vi "E_pressure_comparitor.vi"(1 "Vacuum State":bool[](array[boolean])) -> (0 "output array":bool[](array[boolean]))   [LabVIEW 2015]
panel:
  in  "Turbo Status Array":bool[](array[boolean])
  in  "Pressures":dbl[](array[numeric])
  # "Beamline 1"
  # "1"
  # "Beamline 2"
  # "2"
  # "1"
  # "3"
  # "Beamline 3"
  # "2"
  # "4"
  # "LEIL"
  # "5"
  # "3"
  # "6"
  # "Turbo 1"
  # "7"
  # "Turbo 2"
  # "8"
  # "Turbo 3"
  # "Post LEIL"
  # "Micro Ion"
  # "Cryo 1"
  # "Cryo 2"
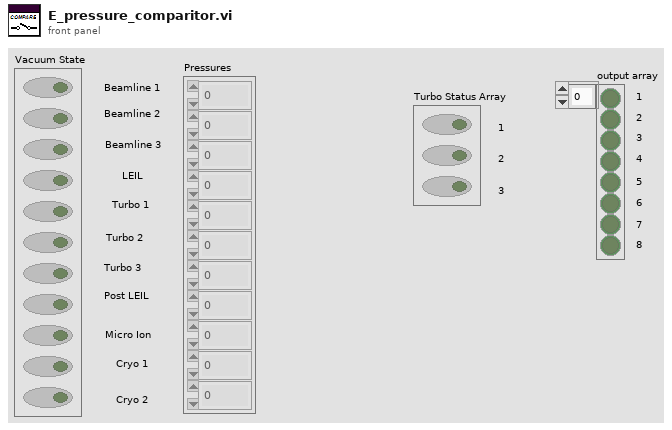
[diagram p1: front panel]
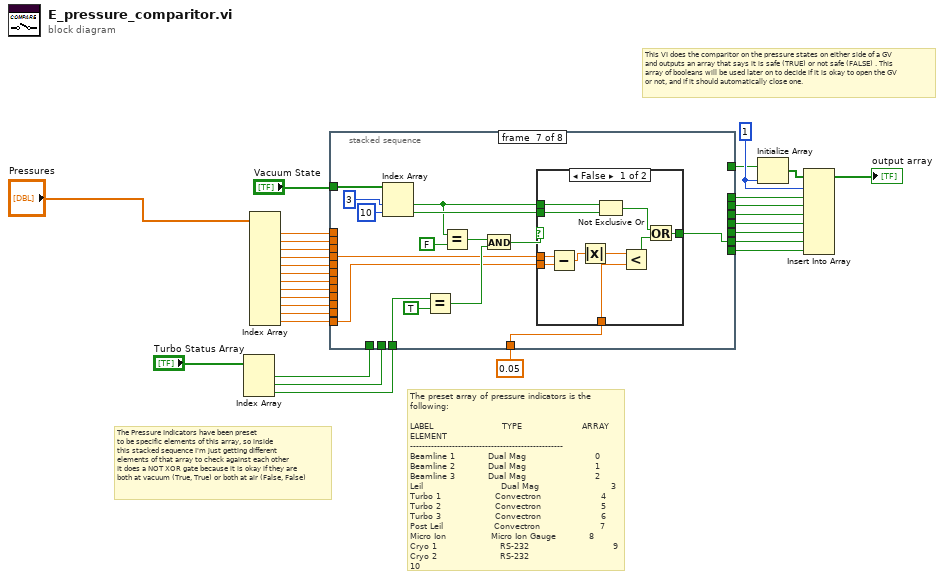
[diagram p0: block diagram]
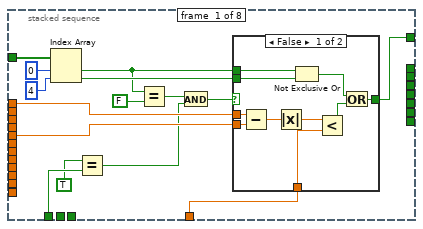
[diagram p2: hidden frame]
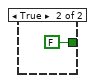
[diagram p3: hidden frame]
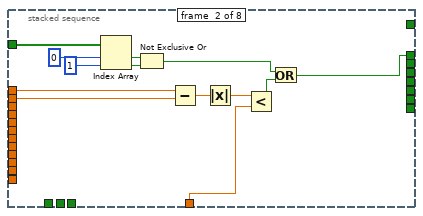
[diagram p4: hidden frame]
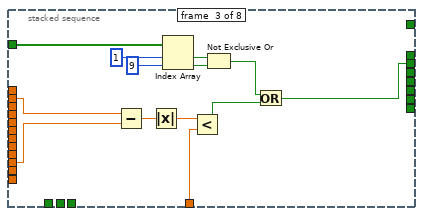
[diagram p5: hidden frame]
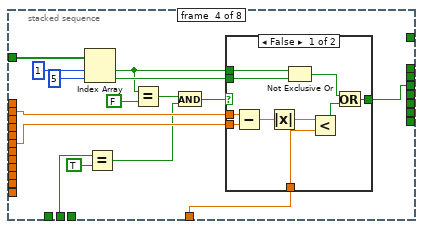
[diagram p6: hidden frame]
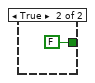
[diagram p7: hidden frame]
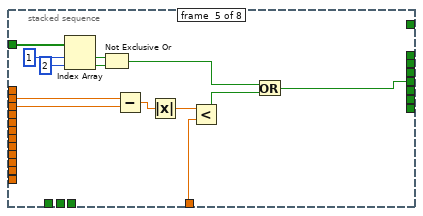
[diagram p8: hidden frame]
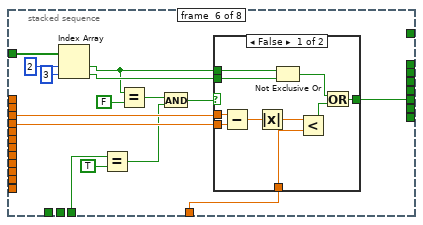
[diagram p9: hidden frame]
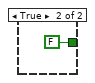
[diagram p10: hidden frame]
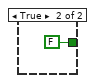
[diagram p11: hidden frame]
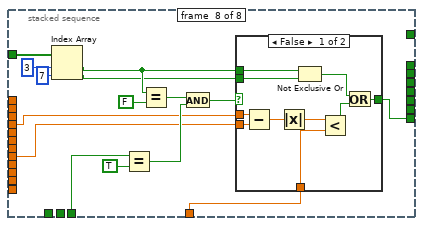
[diagram p12: hidden frame]
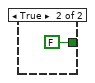
[diagram p13: hidden frame]
diagram:
  w22 = 1 ("dimension size")
  # "The preset array of pressure indicators is the following:\n\nLABEL                       TYPE                    ARRAY ELEMENT\n---------------------------------------------------\nBeamline 1           Dual Mag                       0\nBeamline 2           Dual Mag                       1\nBeamline 3           Dual Mag                       2\nLeil                          Dual Mag                        3\nTurbo 1                  Convectron                    4\nTurbo 2                  Convectron                    5\nTurbo 3                  Convectron                    6\nPost Leil                 Convectron                    7\nMicro Ion               Micro Ion Gauge           8\nCryo 1                     RS-232                            9\nCryo 2                     RS-232                            10"
  # "The Pressure Indicators have been preset\nto be specific elements of this array, so inside \nthis stacked sequence I'm just getting different\nelements of that array to check against each other \nIt does a NOT XOR gate because it is okay if they are \nboth at vacuum (True, True) or both at air (False, False)"
  # "This VI does the comparitor on the pressure states on either side of a GV\nand outputs an array that says it is safe (TRUE) or not safe (FALSE) . This\narray of booleans will be used later on to decide if it is okay to open the GV\nor not, and if it should automatically close one."
  n1 = Index Array(array="Turbo Status Array") -> (element #1=w4:bool, element #2=w3:bool, element #3=w2:bool)  [unwired: 3 in]
  n2 = Index Array(array="Pressures") -> (element #1=w17:dbl, element #2=w16:dbl, element #3=w15:dbl, element #4=w14:dbl, element #5=w13:dbl, element #6=w12:dbl, element #7=w11:dbl, element #8=w10:dbl, element #9=w9:dbl, element #10=w8:dbl, element #11=w7:dbl, element #12=w1:dbl)  [unwired: 12 in]
  n3 = stacked-sequence {
    tunnel: [_ w57 _ _ _ _ _ _] -> w29
    tunnel: [_ _ w70 _ _ _ _ _] -> w28
    tunnel: [_ _ _ w93 _ _ _ _] -> w27
    tunnel: [_ _ _ _ w109 _ _ _] -> w26
    tunnel: [_ _ _ _ _ w133 _ _] -> w25
    tunnel: [_ _ _ _ _ _ w151 _] -> w24
    tunnel: [_ _ _ _ _ _ _ w180] -> w23
    tunnel: [w36 _ _ _ _ _ _ _] -> w21
    tunnel: "Vacuum State" -> [w42 w65 w78 w95 w117 w134 w160 w186]
    tunnel: w17 -> [w41 w61 _ _ _ _ _ _]
    tunnel: w16 -> [_ w60 w74 w92 w112 _ _ _]
    tunnel: w15 -> [_ _ _ _ w111 w131 _ _]
    tunnel: w14 -> [_ _ _ _ _ w130 w153 w176]
    tunnel: w13 -> [w40 _ _ _ _ _ _ _]
    tunnel: w12 -> [_ _ _ w91 _ _ _ _]
    tunnel: w11 -> [_ _ _ _ _ _ _ _]
    tunnel: w10 -> [_ _ _ _ _ _ _ w175]
    tunnel: w9 -> [_ _ _ _ _ _ _ _]
    tunnel: w8 -> [_ _ w73 _ _ _ _ _]
    tunnel: w7 -> [_ _ _ _ _ _ _ _]
    tunnel: 0.05 ("y") -> [w39 w59 w72 w94 w113 w132 w154 w179]
    tunnel: w4 -> [w38 _ _ _ _ _ _ _]
    tunnel: w3 -> [_ _ _ w83 _ _ _ _]
    tunnel: w2 -> [_ _ _ _ _ w124 w152 w174]
    tunnel: w1 -> [_ _ _ _ _ _ w148 _]
    frame #0 {
      n4 = Index Array(array=w42, index #1=0 ("index"), index #2=4 ("index")) -> (element #1=w35:bool, element #2=w45:bool)
      n5 = Equal?(x=TRUE ("y"), y=w38) -> (x = y?=w32:bool)
      n6 = Equal?(x=w35, y=FALSE) -> (x = y?=w33:bool)
      n7 = And(x=w33, y=w32) -> (x .and. y?=w31:bool)
      n8 = case shown="False" w31 {
        tunnel: w35 -> [w55 _]
        tunnel: w45 -> [w54 _]
        tunnel: w41 -> [w53 _]
        tunnel: w40 -> [w52 _]
        tunnel: [w47 FALSE] -> w36
        tunnel: w39 -> [w46 _]
        frame False {
          n9 = Subtract(x=w53, y=w52) -> (x-y=w51:dbl)
          n10 = Absolute Value(x=w51) -> (abs(x)=w50:dbl)
          n11 = Not Exclusive Or(1:w54, 2:w55) -> (0:w48:bool)
          n12 = Less?(x=w50, y=w46) -> (x < y?=w49:bool)
          n13 = Or(x=w48, y=w49) -> (x .or. y?=w47:bool)
        }
        frame True {
        }
      }
    }
    frame #1 {
      n14 = Index Array(array=w65, index #1=0 ("index"), index #2=1 ("index")) -> (element #1=w69:bool, element #2=w68:bool)
      n15 = Not Exclusive Or(1:w68, 2:w69) -> (0:w58:bool)
      n16 = Subtract(x=w61, y=w60) -> (x-y=w64:dbl)
      n17 = Absolute Value(x=w64) -> (abs(x)=w63:dbl)
      n18 = Less?(x=w63, y=w59) -> (x < y?=w62:bool)
      n19 = Or(x=w58, y=w62) -> (x .or. y?=w57:bool)
    }
    frame #2 {
      n20 = Subtract(x=w74, y=w73) -> (x-y=w77:dbl)
      n21 = Absolute Value(x=w77) -> (abs(x)=w76:dbl)
      n22 = Index Array(array=w78, index #1=1 ("index"), index #2=9 ("index")) -> (element #1=w82:bool, element #2=w81:bool)
      n23 = Less?(x=w76, y=w72) -> (x < y?=w75:bool)
      n24 = Not Exclusive Or(1:w81, 2:w82) -> (0:w71:bool)
      n25 = Or(x=w71, y=w75) -> (x .or. y?=w70:bool)
    }
    frame #3 {
      n26 = Index Array(array=w95, index #1=1 ("index"), index #2=5 ("index")) -> (element #1=w86:bool, element #2=w90:bool)
      n27 = Equal?(x=w83, y=TRUE) -> (x = y?=w84:bool)
      n28 = Equal?(x=w86, y=FALSE) -> (x = y?=w88:bool)
      n29 = And(x=w88, y=w84) -> (x .and. y?=w87:bool)
      n30 = case shown="False" w87 {
        tunnel: w86 -> [w107 _]
        tunnel: w90 -> [w106 _]
        tunnel: w92 -> [w105 _]
        tunnel: w91 -> [w104 _]
        tunnel: [w99 FALSE] -> w93
        tunnel: w94 -> [w98 _]
        frame False {
          n31 = Subtract(x=w105, y=w104) -> (x-y=w103:dbl)
          n32 = Absolute Value(x=w103) -> (abs(x)=w102:dbl)
          n33 = Not Exclusive Or(1:w106, 2:w107) -> (0:w100:bool)
          n34 = Less?(x=w102, y=w98) -> (x < y?=w101:bool)
          n35 = Or(x=w100, y=w101) -> (x .or. y?=w99:bool)
        }
        frame True {
        }
      }
    }
    frame #4 {
      n36 = Index Array(array=w117, index #1=1 ("index"), index #2=2 ("index")) -> (element #1=w121:bool, element #2=w120:bool)
      n37 = Not Exclusive Or(1:w120, 2:w121) -> (0:w110:bool)
      n38 = Subtract(x=w112, y=w111) -> (x-y=w116:dbl)
      n39 = Absolute Value(x=w116) -> (abs(x)=w115:dbl)
      n40 = Less?(x=w115, y=w113) -> (x < y?=w114:bool)
      n41 = Or(x=w110, y=w114) -> (x .or. y?=w109:bool)
    }
    frame #5 {
      n42 = Index Array(array=w134, index #1=2 ("index"), index #2=3 ("index")) -> (element #1=w126:bool, element #2=w129:bool)
      n43 = Equal?(x=w124, y=TRUE) -> (x = y?=w123:bool)
      n44 = Equal?(x=w126, y=FALSE) -> (x = y?=w127:bool)
      n45 = And(x=w127, y=w123) -> (x .and. y?=w122:bool)
      n46 = case shown="False" w122 {
        tunnel: w126 -> [w146 _]
        tunnel: w129 -> [w145 _]
        tunnel: w131 -> [w144 _]
        tunnel: w130 -> [w143 _]
        tunnel: [w138 FALSE] -> w133
        tunnel: w132 -> [w137 _]
        frame False {
          n47 = Subtract(x=w144, y=w143) -> (x-y=w142:dbl)
          n48 = Absolute Value(x=w142) -> (abs(x)=w141:dbl)
          n49 = Not Exclusive Or(1:w145, 2:w146) -> (0:w139:bool)
          n50 = Less?(x=w141, y=w137) -> (x < y?=w140:bool)
          n51 = Or(x=w139, y=w140) -> (x .or. y?=w138:bool)
        }
        frame True {
        }
      }
    }
    frame #6 {
      n52 = Index Array(array=w160, index #1=3 ("index"), index #2=10 ("index")) -> (element #1=w149:bool, element #2=w150:bool)
      n53 = Equal?(x=w152, y=TRUE) -> (x = y?=w156:bool)
      n54 = Equal?(x=w149, y=FALSE) -> (x = y?=w158:bool)
      n55 = And(x=w158, y=w156) -> (x .and. y?=w155:bool)
      n56 = case shown="False" w155 {
        tunnel: w149 -> [w172 _]
        tunnel: w150 -> [w171 _]
        tunnel: w153 -> [w170 _]
        tunnel: w148 -> [w169 _]
        tunnel: [w164 FALSE] -> w151
        tunnel: w154 -> [w163 _]
        frame False {
          n57 = Subtract(x=w170, y=w169) -> (x-y=w168:dbl)
          n58 = Absolute Value(x=w168) -> (abs(x)=w167:dbl)
          n59 = Not Exclusive Or(1:w171, 2:w172) -> (0:w165:bool)
          n60 = Less?(x=w167, y=w163) -> (x < y?=w166:bool)
          n61 = Or(x=w165, y=w166) -> (x .or. y?=w164:bool)
        }
        frame True {
        }
      }
    }
    frame #7 {
      n62 = Index Array(array=w186, index #1=3 ("index"), index #2=7 ("index")) -> (element #1=w178:bool, element #2=w177:bool)
      n63 = Equal?(x=w174, y=TRUE) -> (x = y?=w182:bool)
      n64 = Equal?(x=w178, y=FALSE) -> (x = y?=w184:bool)
      n65 = And(x=w184, y=w182) -> (x .and. y?=w181:bool)
      n66 = case shown="False" w181 {
        tunnel: w178 -> [w198 _]
        tunnel: w177 -> [w197 _]
        tunnel: w176 -> [w196 _]
        tunnel: w175 -> [w195 _]
        tunnel: [w190 FALSE] -> w180
        tunnel: w179 -> [w189 _]
        frame False {
          n67 = Subtract(x=w196, y=w195) -> (x-y=w194:dbl)
          n68 = Absolute Value(x=w194) -> (abs(x)=w193:dbl)
          n69 = Not Exclusive Or(1:w197, 2:w198) -> (0:w191:bool)
          n70 = Less?(x=w193, y=w189) -> (x < y?=w192:bool)
          n71 = Or(x=w191, y=w192) -> (x .or. y?=w190:bool)
        }
        frame True {
        }
      }
    }
  }
  n72 = Initialize Array(w21, w22) -> (w30:bool[])
  n73 = Insert Into Array(array=w30, index=w22, new element #1=w29, new element #2=w28, new element #3=w27, new element #4=w26, new element #5=w25, new element #6=w24, new element #7=w23) -> (→"output array":bool[])
